vi "Warning Light.vi"() -> ()   [LabVIEW 2017]
doc: "Use this template to simulate the generation and display of data.\nNote: LabVIEW enables automatic error handling by default for VIs you create from this template."
uses:
  Instance           1 27Saved   GenerateDisplay.vit .vi
  <vilib>/express/express shared/transition.llb/Dynamic To Waveform Array.vi
  <vilib>/express/express arith-compare/Formula/Block/exnFormulaBlock how many pts in the wave.vi
  <vilib>/express/express shared/ex_Modify Signal Name.vi
  <vilib>/express/express shared/transition.llb/Waveform Array To Dynamic.vi
  <vilib>/express/express arith-compare/Formula/XNode/ExpressFormulaBlockNode.xnode
panel:
  out "Peak to Peak":dbl
  out "Warning":bool
  out "Filtered Signal":dynamicdata(graph)
  out "Unfiltered Signal":dynamicdata(graph)
  in  "stop":bool
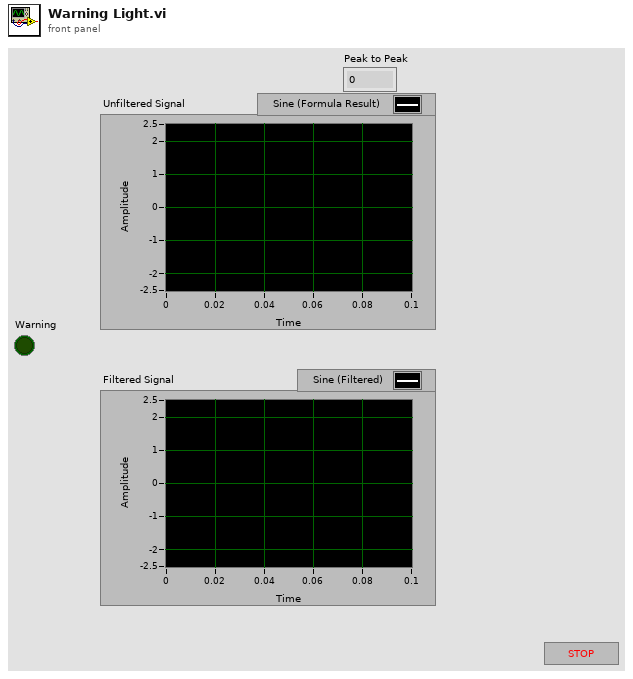
[diagram p1: front panel]
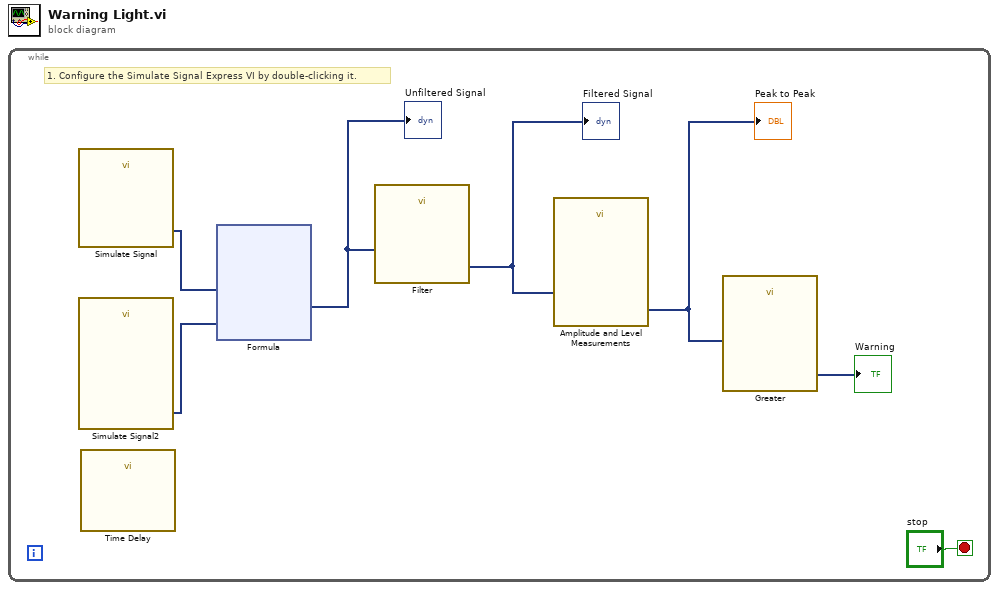
[diagram p0: block diagram]
diagram:
  n1 = while {
    stop <- "stop" stop-if-true
    # "1. Configure the Simulate Signal Express VI by double-clicking it."
    n2 = call "Simulate Signal"() -> ("Sine"=w6:dynamicdata)  [unwired: 14 in, 1 out]
    n3 = call "Simulate Signal2"() -> ("60 Hz and Noise"=w5:dynamicdata)  [unwired: 14 in, 1 out]
    n4 = call "Time Delay"() -> ()  [unwired: 11 in, 1 out]
    n5 = xnode "Formula"("Sine"=w6, "60Hz and Noise"=w5) -> ("Result"=w4:dynamicdata)  [unwired: 1 in, 1 out]
    "Unfiltered Signal" <- w4
    n6 = call "Filter"("Signal"=w4) -> ("Filtered Signal"=w3:dynamicdata)  [unwired: 9 in, 1 out]
    "Filtered Signal" <- w3
    n7 = call "Amplitude and Level Measurements"("Signals"=w3) -> ("Peak to Peak"=w2:dynamicdata)  [unwired: 13 in, 1 out]
    "Peak to Peak" <- w2
    n8 = call "Greater"("Operand 1"=w2) -> ("Result"=→"Warning":dynamicdata)  [unwired: 9 in, 1 out]
  }
